vi "Adler32.vi"(1 "Modulus?":bool=TRUE, 2 "String":string) -> (0 "Checksum":u32)   [LabVIEW 2009]
panel:
  out "B":u16
  out "A":u16
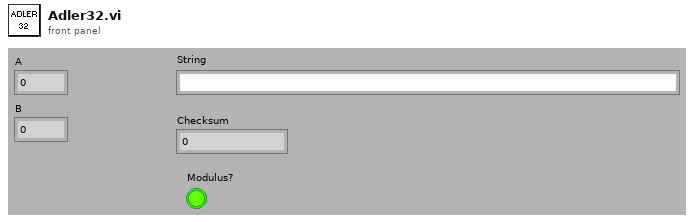
[diagram p1: front panel]
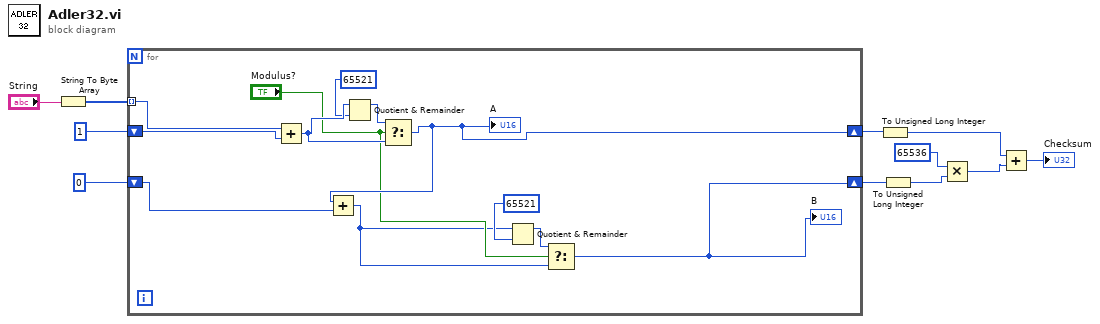
[diagram p0: block diagram]
diagram:
  n1 = String To Byte Array(string="String") -> (unsigned byte array=w10:u8[])
  n2 = for {
    tunnel: w10 -> [w23] mode=indexing
    shift-right: [w17] -> w6
    shift-left: u16 1 ("A") -> [w22]
    shift-right: [w12] -> w7
    shift-left: u16 0 ("A") -> [w21]
    n3 = Add(x=w23, y=w22) -> (x+y=w20:u16)
    n4 = Quotient & Remainder(x=w20, y=u16 65521) -> (x-y*floor(x/y)=w18:u16)  [unwired: 1 out]
    n5 = Select(t=w18, s="Modulus?", f=w20) -> (s? t:f=w17:u16)
    "A" <- w17
    n6 = Add(x=w17, y=w21) -> (x+y=w13:u16)
    n7 = Quotient & Remainder(x=w13, y=u16 65521) -> (x-y*floor(x/y)=w16:u16)  [unwired: 1 out]
    n8 = Select(t=w16, s="Modulus?", f=w13) -> (s? t:f=w12:u16)
    "B" <- w12
  }
  n9 = To Unsigned Long Integer(number=w6) -> (unsigned 32bit integer=w1:u32)
  n10 = To Unsigned Long Integer(number=w7) -> (unsigned 32bit integer=w3:u32)
  n11 = Multiply(x=u32 65536 ("y"), y=w3) -> (x*y=w2:u32)
  n12 = Add(x=w1, y=w2) -> (x+y=→"Checksum":u32)
